vi "run.search.vi"(8 "error in":errorcluster, 11 "Client in":refnum<class "Client.lvclass">) -> (0 "error out":errorcluster, 3 "Client out":refnum<class "Client.lvclass">)   [LabVIEW 2020, in "Client.lvclass"]
doc: "Searches for runs matching the given text, label, property, run number, and/or start/end time filters and returns a handle list of matches."
uses:
  Client.lvclass
  client.lvlib
panel:
  out "out_list out":i32
  out "out_count out":u32
  in  "out_count":u32
  in  "out_list":i32
  in  "has_end_before":bool
  in  "end_before_ms":dbl
  in  "has_start_after":bool
  in  "start_after_ms":dbl
  in  "run_number":u32
  in  "property_value":string
  in  "property_key":string
  in  "label":string
  in  "search_text":string
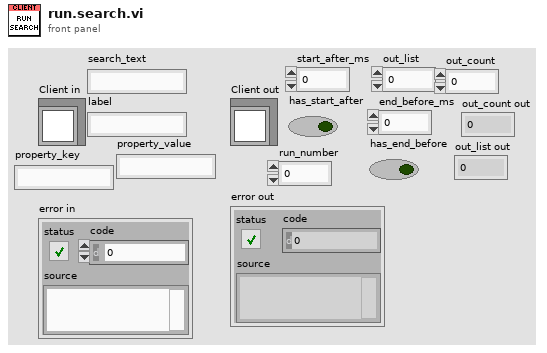
[diagram p1: front panel]
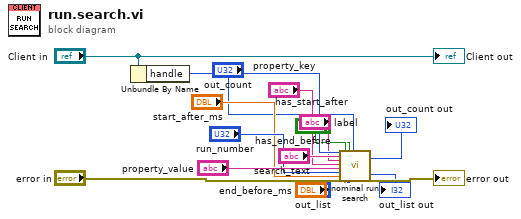
[diagram p0: block diagram]
diagram:
  n1 = Unbundle By Name("Client in") -> ("handle"=w15:i32)
  n2 = call "nominal run search.vi"("client"=w15, "search_text"="search_text", "label"="label", "property_key"="property_key", "property_value"="property_value", "run_number"="run_number", "start_after_ms"="start_after_ms", "error in (no error)"="error in", "has_start_after"="has_start_after", "end_before_ms"="end_before_ms", "has_end_before"="has_end_before", "out_list"="out_list", "out_count"="out_count") -> ("out_count out"=→"out_count out":u32, "out_list out"=→"out_list out":i32, "error out"=→"error out":errorcluster)  [unwired: 11 in, 1 out]
  "Client out" <- "Client in"
